vi "周期设置_多参数.vi"() -> ()   [LabVIEW 2016, in "斯坦道多参数.lvlib"]
uses:
  <vilib>/Utility/miscctls.llb/LVPointTypeDef.ctl
  <vilib>/ptbypt/NI_PtbyPt.lvlib
  <vilib>/Utility/config.llb/NI_LVConfig.lvlib
panel:
  in  "运行周期":T1
  # "运行模式："
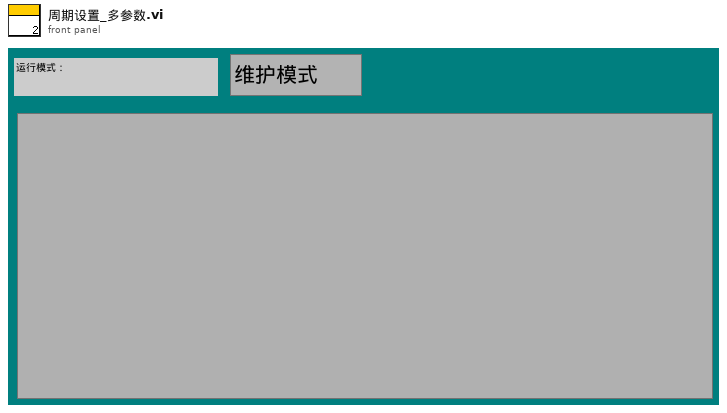
[diagram p1: front panel]
types:
  T1 = cluster{"运行模式":enum16{"维护模式", "常规模式", "应急模式", "质控模式"}, "24H周期设置":bool[]}
  T2 = typedef "LVPointTypeDef.ctl" = cluster{"Horizontal":i16, "Vertical":i16}
  T3 = typedef "LVDateTimeRec.ctl" = cluster{"秒数的小数部分":dbl, "秒":i32, "分":i32, "时":i32, "日":i32, "月":i32, "年":i32, "天数（周）":i32, "天数（年）":i32, "DST":i32}
  T4 = typedef "NI_LVConfig.lvlib/Config Data RefNum.ctl" = refnum<k1>
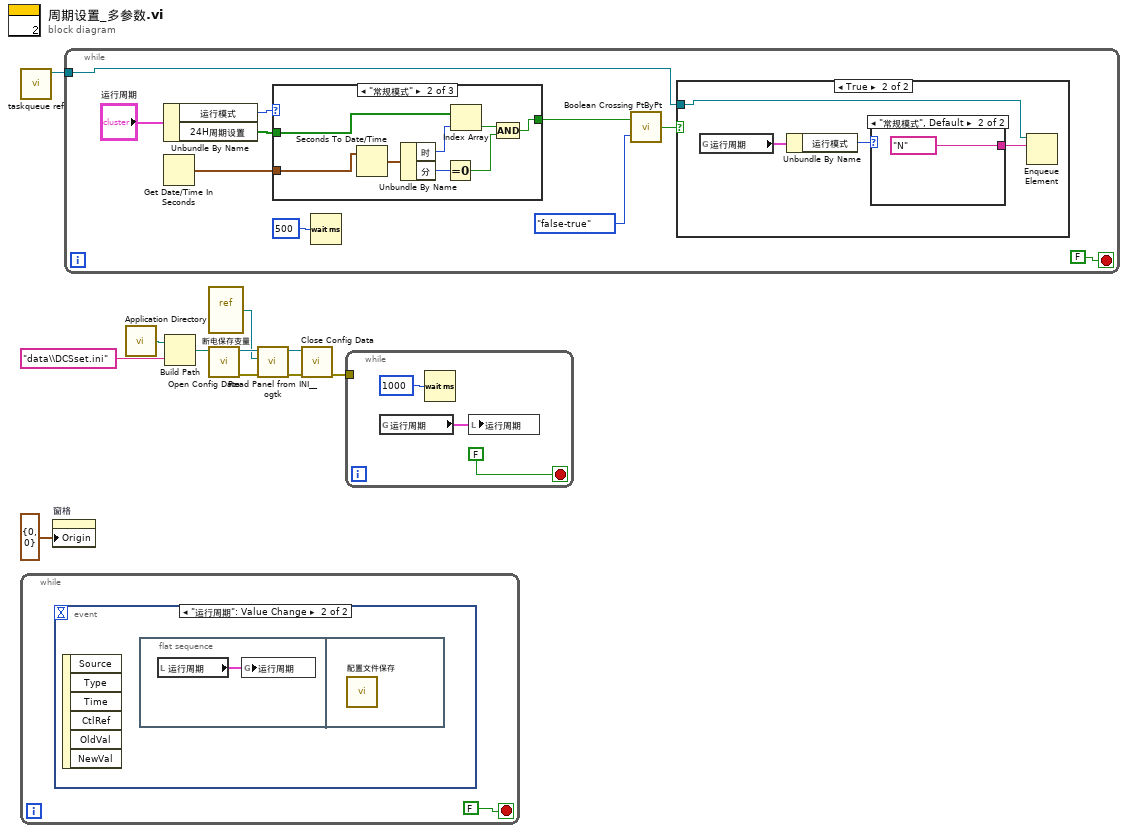
[diagram p0: block diagram]
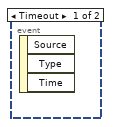
[diagram p2: hidden frame]
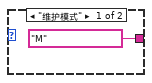
[diagram p4: hidden frame]
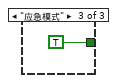
[diagram p6: hidden frame]
diagram:
  n1 = call "taskqueue ref.vi"() -> ("队列输出"=w4:refnum<queue>)  [unwired: 10 in, 1 out]
  n2 = while {
    stop <- FALSE stop-if-true
    n3 = event shown="[1] \"运行周期\": Value Change" {
      selector: _ -> [_ _]
      dyn-events: _ -> [_ _]
      timeout: _ -> [_ _]
      event Timeout {
        n4 = event-data() -> ()  [unwired: 1 in, 3 out]
      }
      event "运行周期": Value Change {
        n5 = event-data() -> ()  [unwired: 1 in, 6 out]
        n6 = flat-sequence {
          frame #0 {
            n7 = local read "运行周期"() -> (w13:T1)
            n8 = global write "断电保存变量.vi" "运行周期"(w13) -> ()
          }
          frame #1 {
            n9 = call "配置文件保存.vi"() -> ()  [unwired: 12 in]
          }
        }
      }
    }
  }
  n10 = property on="窗格" class="Pane"("Origin"=T2 {"Horizontal"=0, "Vertical"=0} ("原点")) -> ()  [unwired: 2 in, 2 out]
  n11 = while {
    tunnel: w4 -> [w14]
    stop <- FALSE stop-if-true
    n12 = Unbundle By Name("运行周期") -> ("运行模式"=w18:enum16{"维护模式", "常规模式", "应急模式", "质控模式"}, "24H周期设置"=w19:bool[])
    n13 = Get Date/Time In Seconds() -> (seconds since 1Jan1904=w23:timestamp)
    n14 = case shown="\"常规模式\"" w18 {
      tunnel: w23 -> [_ w37 _]
      tunnel: w19 -> [_ w34 _]
      tunnel: [_ w30 TRUE] -> w17
      frame "维护模式", Default {
      }
      frame "常规模式" {
        n15 = Seconds To Date/Time(time stamp (now)=w37) -> (date time rec=w36:T3)  [unwired: 1 in]
        n16 = Unbundle By Name(w36) -> ("时"=w35:i32, "分"=w33:i32)
        n17 = Equal To 0?(x=w33) -> (x = 0?=w31:bool)
        n18 = Index Array(array=w34, index=w35) -> (element=w32:bool)
        n19 = Compound Arithmetic op=AND ("复合运算")(w32, w31) -> (w30:bool)
      }
      frame "应急模式" {
      }
    }
    n20 = Wait (ms)(milliseconds to wait=u32 500 ("等待时间（毫秒）")) -> ()  [unwired: 1 out]
    n21 = call <vilib>:"Boolean Crossing PtByPt.vi"("direction"=enum16{"either", "false-true", "true-false"}."false-true", "input"=w17) -> ("crossing"=w15:bool)  [unwired: 1 in]
    n22 = case shown="True" w15 {
      tunnel: w14 -> [_ w25]
      frame False {
      }
      frame True {
        n23 = global read "断电保存变量.vi" "运行周期"() -> (w27:T1)
        n24 = Unbundle By Name(w27) -> ("运行模式"=w26:enum16{"维护模式", "常规模式", "应急模式", "质控模式"})
        n25 = case shown="\"常规模式\", Default" w26 {
          tunnel: ["M" ("数据标记表") "N" ("数据标记表")] -> w24
          frame "维护模式" {
          }
          frame "常规模式", Default {
          }
        }
        n26 = Enqueue Element(queue=w25, element=w24) -> ()  [unwired: 2 in, 3 out]
      }
    }
  }
  n27 = call <vilib>:"Application Directory.vi"() -> ("Application Directory"=w3:path)
  n28 = Build Path(base path=w3, name or relative path="data\\DCSset.ini" ("名称或相对路径")) -> (appended path=w1:path)
  n29 = vi-ref "断电保存变量.vi"() -> (w6:refnum<vi>)
  n30 = call <vilib>:"Open Config Data.vi"("configuration file path"=w1) -> ("error out"=w9:errorcluster, "refnum"=w10:T4)  [unwired: 8 in, 1 out]
  n31 = call <userlib>:"Read Panel from INI__ogtk.vi"("error in (no error)"=w9, "VI ref"=w6, "refnum"=w10) -> ("error out"=w7:errorcluster, "refnum out"=w8:T4)  [unwired: 7 in]
  n32 = call <vilib>:"Close Config Data.vi"("error in (no error)"=w7, "refnum"=w8) -> ("error out"=w5:errorcluster)  [unwired: 8 in, 1 out]
  n33 = while {
    tunnel: w5 -> [_]
    stop <- FALSE stop-if-true
    n34 = global read "断电保存变量.vi" "运行周期"() -> (w39:T1)
    n35 = Wait (ms)(milliseconds to wait=u32 1000 ("等待时间（毫秒）")) -> ()  [unwired: 1 out]
    n36 = local write "运行周期"(w39) -> ()
  }
